vi "6-17.vi"() -> ()   [LabVIEW 2017]
panel:
  in  "stop":bool
  out "Waveform Chart":dbl(graph)
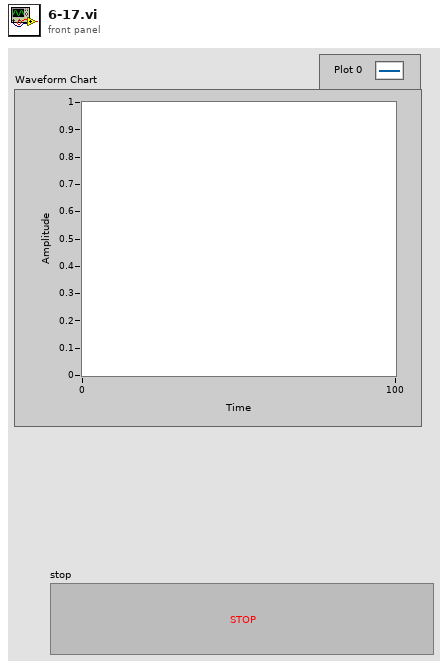
[diagram p1: front panel]
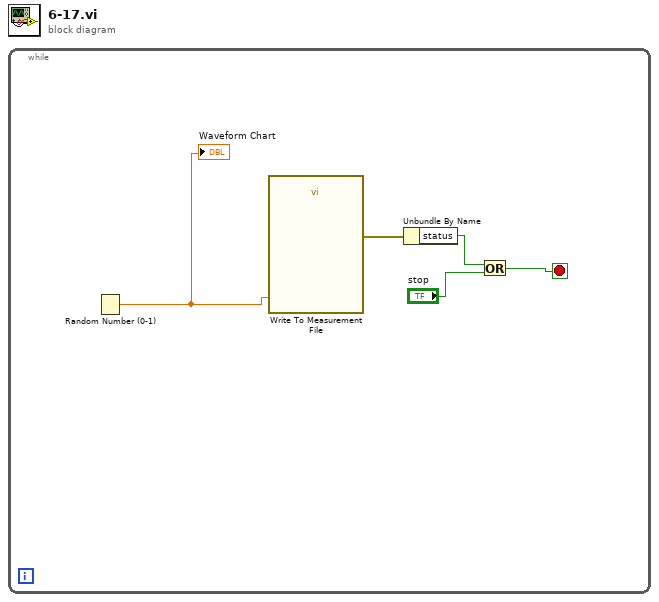
[diagram p0: block diagram]
diagram:
  n1 = while {
    stop <- w1 stop-if-true
    n2 = Random Number (0-1)() -> (number: 0 to 1=w5:dbl)
    "Waveform Chart" <- w5
    n3 = call "Write To Measurement File"("Signals"=w5) -> ("error out"=w4:errorcluster)  [unwired: 16 in, 2 out]
    n4 = Unbundle By Name(w4) -> ("status"=w3:bool)
    n5 = Or(x=w3, y="stop") -> (x .or. y?=w1:bool)
  }
